vi "Create Plugin Bundle.vi"(7 "ID":i32, 8 "error in (no error)":errorcluster, 9 "Transfer Groups":refnum<class "Transfer Group.lvclass">[](array[class]), 10 "Timing":refnum<class "Timing.lvclass">, 11 "Scheduler Plugin Bundle in":refnum<class "Scheduler Plugin Bundle.lvclass">) -> (0 "error out":errorcluster, 3 "Scheduler Plugin Bundle out":refnum<class "Scheduler Plugin Bundle.lvclass">)   [LabVIEW 2017, in "DSF Core.lvlib" / "Scheduler Plugin Bundle.lvclass"]
uses:
  Scheduler Plugin Bundle.lvclass
  Timing/Timing.lvclass
  Transfer Group/Transfer Group.lvclass
  Scheduler Plugin Bundle.lvclass/Scheduler Plugin Bundle.ctl
  Scheduler Transfer Group Bundle.lvclass
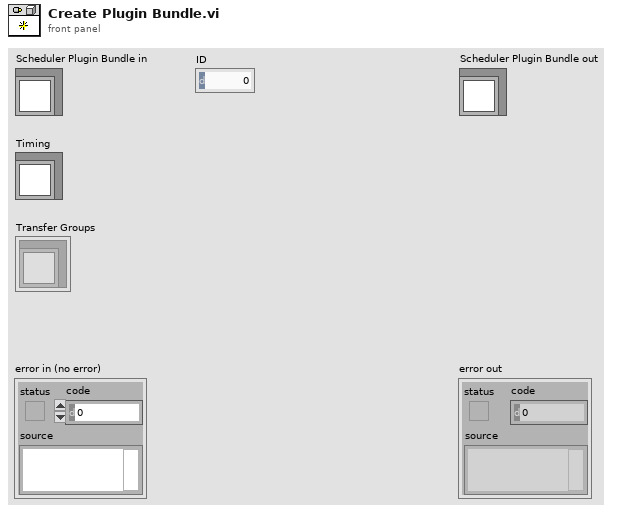
[diagram p1: front panel]
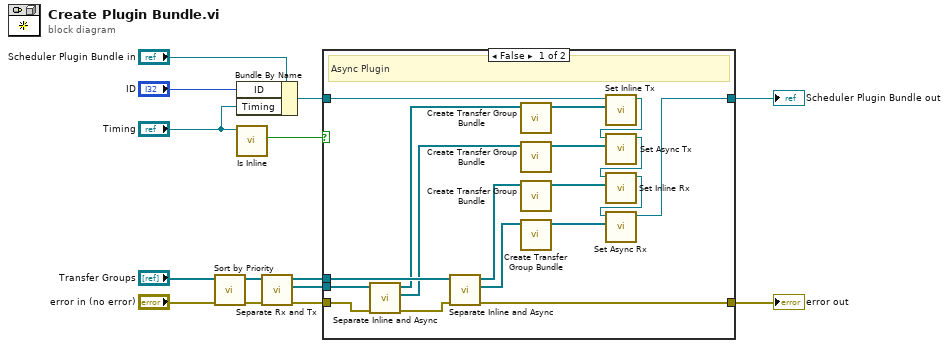
[diagram p0: block diagram]
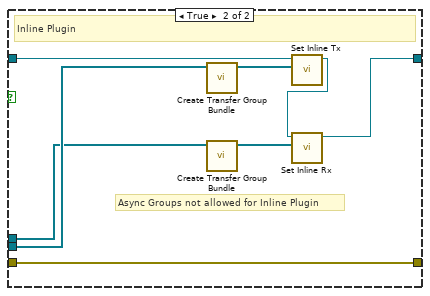
[diagram p2: hidden frame]
diagram:
  n1 = call "Sort by Priority.vi"("error in (no error)"="error in (no error)", "Transfer Groups"="Transfer Groups") -> ("error out"=w12:errorcluster, "sorted Transfer Groups"=w11:refnum<class "Transfer Group.lvclass">[])  [unwired: 8 in]
  n2 = Bundle By Name(cluster="Scheduler Plugin Bundle in", "ID"="ID", "Timing"="Timing") -> (w5:refnum<class "Scheduler Plugin Bundle.lvclass">)
  n3 = call "Is Inline.vi"("Timing in"="Timing") -> ("inline?"=w7:bool)  [unwired: 9 in, 1 out]
  n4 = call "Separate Rx and Tx.vi"("error in (no error)"=w12, "Transfer Groups"=w11) -> ("error out"=w10:errorcluster, "Tx Transfer Groups"=w9:refnum<class "Transfer Group.lvclass">[], "Rx Transfer Groups"=w8:refnum<class "Transfer Group.lvclass">[])  [unwired: 7 in]
  n5 = case shown="False" w7 {
    tunnel: w10 -> [w32 w38]
    tunnel: w9 -> [w31 w40]
    tunnel: w8 -> [w30 w39]
    tunnel: [w28 w38] -> w1
    tunnel: w5 -> [w16 w33]
    tunnel: [w15 w34] -> w3
    frame False {
      # "Async Plugin"
      n6 = call "Separate Inline and Async.vi"("error in (no error)"=w32, "Transfer Groups"=w31) -> ("error out"=w29:errorcluster, "Async Transfer Groups"=w26:refnum<class "Transfer Group.lvclass">[], "Inline Transfer Groups"=w27:refnum<class "Transfer Group.lvclass">[])  [unwired: 7 in]
      n7 = call "Separate Inline and Async.vi"("error in (no error)"=w29, "Transfer Groups"=w30) -> ("error out"=w28:errorcluster, "Async Transfer Groups"=w24:refnum<class "Transfer Group.lvclass">[], "Inline Transfer Groups"=w25:refnum<class "Transfer Group.lvclass">[])  [unwired: 7 in]
      n8 = call "Create Transfer Group Bundle.vi"("Transfer Groups"=w27) -> ("Transfer Group Bundles"=w23:refnum<class "Scheduler Transfer Group Bundle.lvclass">[])  [unwired: 10 in]
      n9 = call "Create Transfer Group Bundle.vi"("Transfer Groups"=w26) -> ("Transfer Group Bundles"=w22:refnum<class "Scheduler Transfer Group Bundle.lvclass">[])  [unwired: 10 in]
      n10 = call "Create Transfer Group Bundle.vi"("Transfer Groups"=w25) -> ("Transfer Group Bundles"=w21:refnum<class "Scheduler Transfer Group Bundle.lvclass">[])  [unwired: 10 in]
      n11 = call "Create Transfer Group Bundle.vi"("Transfer Groups"=w24) -> ("Transfer Group Bundles"=w20:refnum<class "Scheduler Transfer Group Bundle.lvclass">[])  [unwired: 10 in]
      n12 = call "Set Inline Tx.vi"("Inline Tx"=w23, "Scheduler Plugin Bundle in"=w16) -> ("Scheduler Plugin Bundle out"=w19:refnum<class "Scheduler Plugin Bundle.lvclass">)  [unwired: 9 in]
      n13 = call "Set Async Tx.vi"("Async Tx"=w22, "Scheduler Plugin Bundle in"=w19) -> ("Scheduler Plugin Bundle out"=w18:refnum<class "Scheduler Plugin Bundle.lvclass">)  [unwired: 9 in]
      n14 = call "Set Inline Rx.vi"("Inline Rx"=w21, "Scheduler Plugin Bundle in"=w18) -> ("Scheduler Plugin Bundle out"=w17:refnum<class "Scheduler Plugin Bundle.lvclass">)  [unwired: 9 in]
      n15 = call "Set Async Rx.vi"("Async Rx"=w20, "Scheduler Plugin Bundle in"=w17) -> ("Scheduler Plugin Bundle out"=w15:refnum<class "Scheduler Plugin Bundle.lvclass">)  [unwired: 9 in]
    }
    frame True {
      # "Async Groups not allowed for Inline Plugin"
      # "Inline Plugin"
      n16 = call "Create Transfer Group Bundle.vi"("Transfer Groups"=w40) -> ("Transfer Group Bundles"=w37:refnum<class "Scheduler Transfer Group Bundle.lvclass">[])  [unwired: 10 in]
      n17 = call "Create Transfer Group Bundle.vi"("Transfer Groups"=w39) -> ("Transfer Group Bundles"=w36:refnum<class "Scheduler Transfer Group Bundle.lvclass">[])  [unwired: 10 in]
      n18 = call "Set Inline Tx.vi"("Inline Tx"=w37, "Scheduler Plugin Bundle in"=w33) -> ("Scheduler Plugin Bundle out"=w35:refnum<class "Scheduler Plugin Bundle.lvclass">)  [unwired: 9 in]
      n19 = call "Set Inline Rx.vi"("Inline Rx"=w36, "Scheduler Plugin Bundle in"=w35) -> ("Scheduler Plugin Bundle out"=w34:refnum<class "Scheduler Plugin Bundle.lvclass">)  [unwired: 9 in]
    }
  }
  "error out" <- w1
  "Scheduler Plugin Bundle out" <- w3
